vi "SineCalculateAndAdvance.vi"(3 "Multiplier advance per cycle":fxp<+/-,32,0>, 4 "FPGA Cycle Parameters In":T2, 5 "FPGA Cycle Counters In":T1) -> (1 "Ramped sine":fxp<+/-,16,12> format="%.28g", 2 "FPGA Cycle Counters Out":T1)   [LabVIEW 2010]
uses:
  FPGA_Typedefs/FPGA Cycle Parameters.ctl
  FPGA_Typedefs/FPGA Cycle Counters.ctl
  <vilib>/rvi/FXPMathLib/FxpSinAndCos/XNode/nifxpmath_SinAndCos.xnode
  <vilib>/rvi/FXPMathLib/FxpSinAndCos/subVIs/nifxpmath_SinAndCos_SimConfig.ctl
  <vilib>/rvi/FXPMathLib/FxpMul/XNode/nifxpmath_Multiplier.xnode
  <vilib>/rvi/FXPMathLib/FxpMul/subVIs/nifxpmath_Mul_SimConfig.ctl
  <vilib>/fxp/LVFixedPointQuantizationPolicyTypeDef.ctl
  <vilib>/fxp/LVFixedPointOverflowPolicyTypeDef.ctl
  <vilib>/rvi/FXPMathLib/FxpAdd/XNode/nifxpmath_Add.xnode
  <vilib>/rvi/FXPMathLib/FxpAdd/subVIs/nifxpmath_Add_SimConfig.ctl
  <vilib>/rvi/FXPMathLib/FxpSinAndCos/simVIs/DllFxpSinAndCosTemp_sub.vi
  <vilib>/rvi/FXPMathLib/FxpMul/simVIs/DllFxpMulTemp_sub.vi
  <vilib>/rvi/FXPMathLib/FxpAdd/simVIs/DllFxpAddTemp_sub.vi
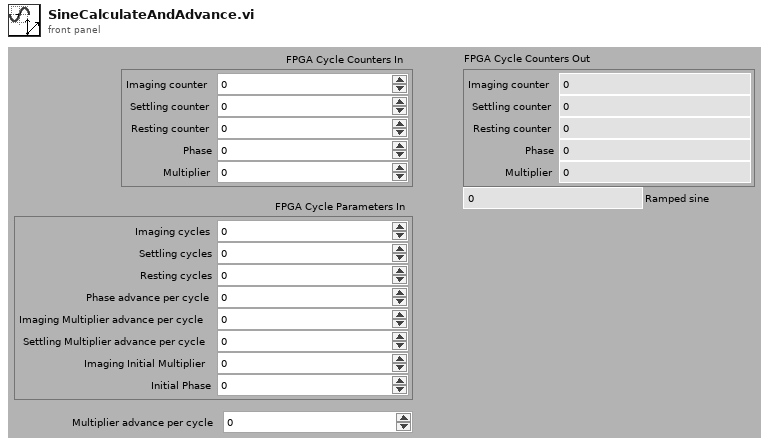
[diagram p1: front panel]
types:
  T1 = typedef "FPGA Cycle Counters.ctl" = cluster{"Imaging counter":i32, "Settling counter":i32, "Resting counter":i32, "Phase":fxp<+,32,1>, "Multiplier":fxp<+/-,43,12>}
  T2 = typedef "FPGA Cycle Parameters.ctl" = cluster{"Imaging cycles":i32, "Settling cycles":i32, "Resting cycles":i32, "Phase advance per cycle":fxp<+,32,0>, "Imaging Multiplier advance per cycle":fxp<+/-,32,0>, "Settling Multiplier advance per cycle":fxp<+/-,32,0>, "Imaging Initial Multiplier":fxp<+/-,43,12>, "Initial Phase":fxp<+,32,1>}
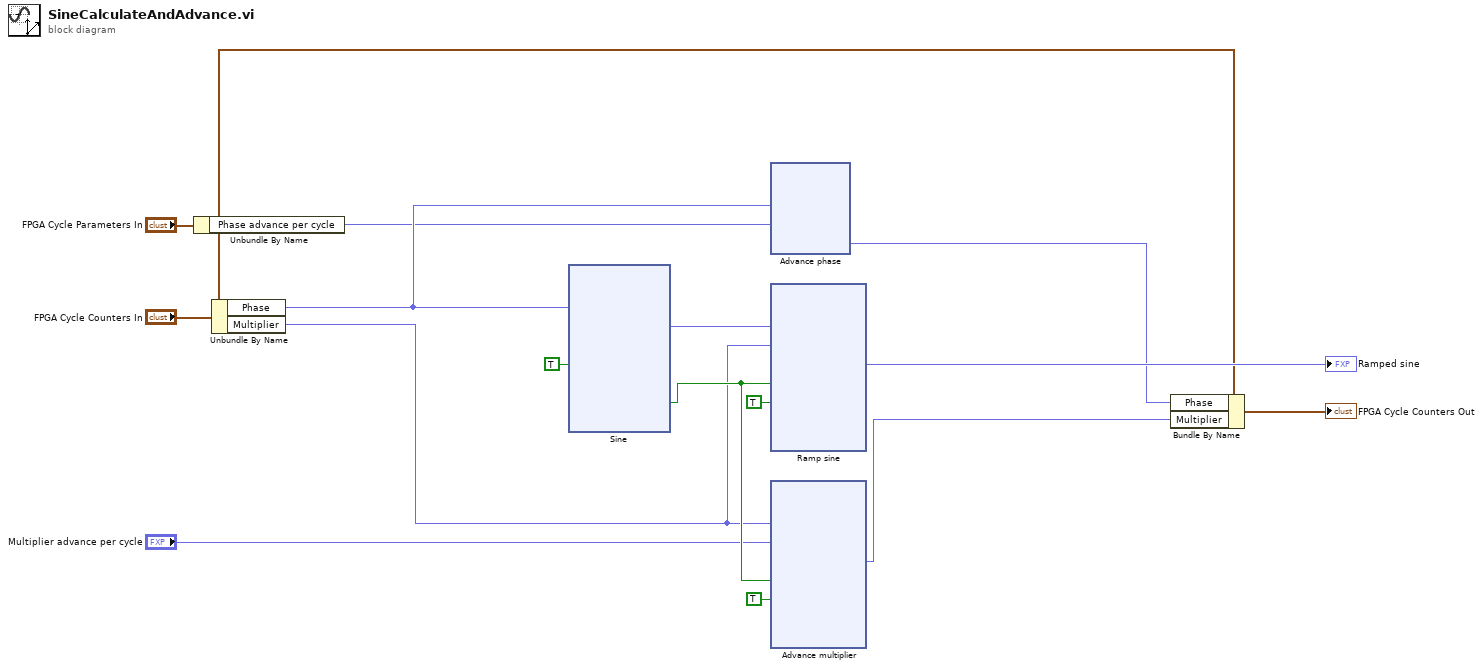
[diagram p0: block diagram]
diagram:
  n1 = Unbundle By Name("FPGA Cycle Parameters In") -> ("Phase advance per cycle"=w5:fxp<+,32,0>)
  n2 = Unbundle By Name("FPGA Cycle Counters In") -> ("Phase"=w7:fxp<+,32,1>, "Multiplier"=w8:fxp<+/-,43,12>)
  n3 = xnode "Sine"("x (pi)"=w7, "input valid"=TRUE) -> ("sin(x)"=w10:fxp<+/-,32,2>, "output valid"=w14:bool)  [unwired: 1 in, 2 out]
  n4 = xnode "Advance phase"("x"=w7, "y"=w5) -> ("x+y"=w3:fxp<+,32,1>)
  n5 = xnode "Ramp sine"("x"=w10, "y"=w8, "input valid"=w14, "ready for output (T)"=TRUE) -> ("x*y"=→"Ramped sine":fxp<+/-,16,12>)  [unwired: 2 out]
  n6 = xnode "Advance multiplier"("x"=w8, "y"="Multiplier advance per cycle", "input valid"=w14, "ready for output (T)"=TRUE) -> ("x+y"=w2:fxp<+/-,43,12>)  [unwired: 2 out]
  n7 = Bundle By Name(cluster="FPGA Cycle Counters In", "Phase"=w3, "Multiplier"=w2) -> (→"FPGA Cycle Counters Out":T1)
